vi "Common_DoesClassExist.vi"(1 "ClassPath":path, 2 "ClassName":string) -> (15 "ClassExists":bool, 16 "llb-class":bool, 17 "llb/LvCLass-Path":path, 18 "LvClassExists":bool)   [LabVIEW 2020]
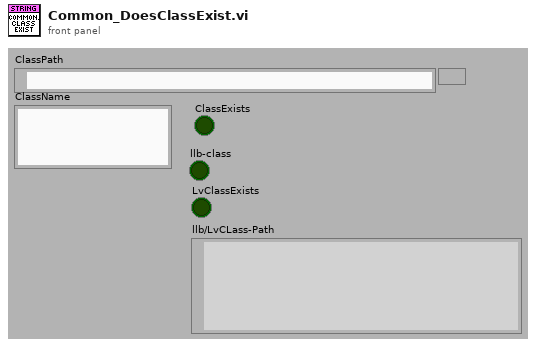
[diagram p1: front panel]
types:
  T1 = typedef "Librarian File Info Out.ctl" = cluster{"creation date":u32, "last mod date":u32, "type":string, "creator":string, "LV version":i32, "size":i32, "top level":bool}
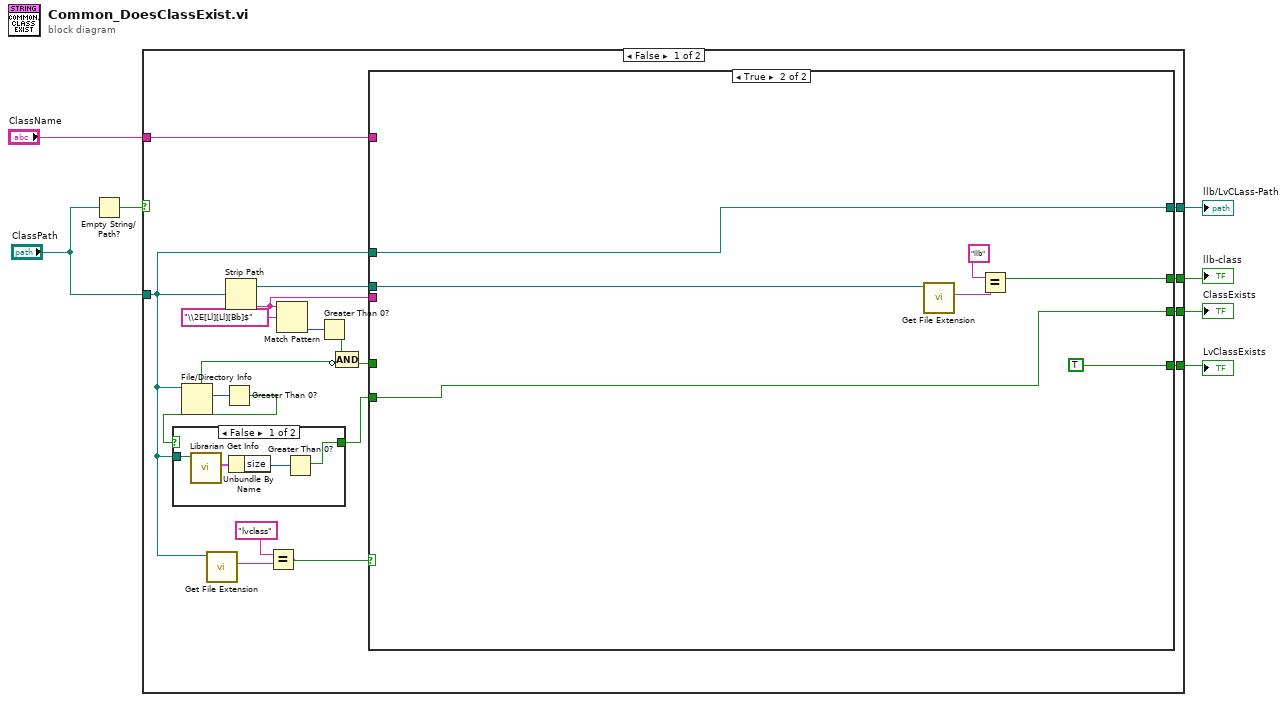
[diagram p0: block diagram]
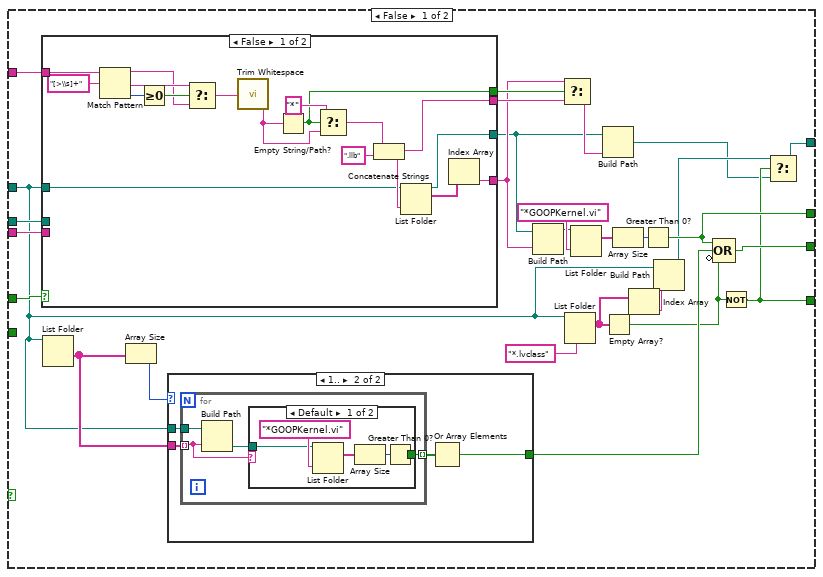
[diagram p3: hidden frame]
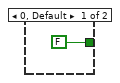
[diagram p4: hidden frame]
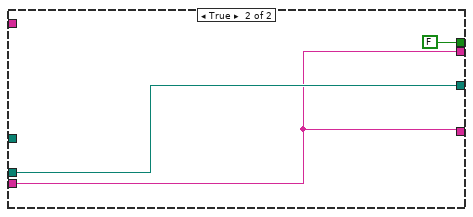
[diagram p6: hidden frame]
diagram:
  n1 = Empty String/Path?(string/path="ClassPath") -> (empty?=w1:bool)
  n2 = case shown="False" w1 {
    tunnel: [w26 _] -> w7
    tunnel: [w25 _] -> w6
    tunnel: "ClassName" -> [w24 _]
    tunnel: [w23 _] -> w4
    tunnel: [w13 _] -> w3
    tunnel: "ClassPath" -> [w11 _]
    frame False {
      n3 = File/Directory Info(path=w11) -> (directory=w10:bool, size=w12:i64)  [unwired: 1 in, 5 out]
      n4 = call <vilib>:"Get File Extension.vi"("file"=w11) -> ("lowercase file extension"=w16:string)  [unwired: 1 in, 9 out]
      n5 = Greater Than 0?(x=w12) -> (x > 0?=w9:bool)
      n6 = case shown="False" w9 {
        selector: w9 -> [_ w31]
        tunnel: w11 -> [w28 _]
        tunnel: [w27 w31] -> w8
        frame False {
          n7 = call <vilib>:"Librarian Get Info.vi"("path"=w28) -> ("file information"=w30:T1)  [unwired: 1 in, 9 out]
          n8 = Unbundle By Name(w30) -> ("size"=w29:i32)
          n9 = Greater Than 0?(x=w29) -> (x > 0?=w27:bool)
        }
        frame True {
        }
      }
      n10 = Strip Path(path=w11) -> (stripped path=w18:path, name=w17:string)
      n11 = Equal?(x="lvclass", y=w16) -> (x = y?=w14:bool)
      n12 = Match Pattern(string=w17, regular expression="\\2E[Ll][Ll][Bb]$") -> (offset past match=w21:i32)  [unwired: 4 out]
      n13 = Greater Than 0?(x=w21) -> (x > 0?=w20:bool)
      n14 = Compound Arithmetic op=AND(w20, invert w10) -> (w19:bool)
      n15 = case shown="True" w14 {
        tunnel: [w40 w95] -> w26
        tunnel: [w32 w93] -> w25
        tunnel: w24 -> [w58 _]
        tunnel: [w48 w96] -> w23
        tunnel: w19 -> [w47 _]
        tunnel: w18 -> [w46 w94]
        tunnel: w17 -> [w45 _]
        tunnel: w11 -> [w36 w93]
        tunnel: [w35 TRUE] -> w13
        tunnel: w8 -> [_ w95]
        frame False {
          n16 = case shown="False" w47 {
            tunnel: w58 -> [w80 _]
            tunnel: [w78 FALSE] -> w57
            tunnel: [w77 w90] -> w56
            tunnel: [w75 w91] -> w42
            tunnel: [w74 w90] -> w50
            tunnel: w36 -> [w73 _]
            tunnel: w46 -> [_ w91]
            tunnel: w45 -> [_ w90]
            frame False {
              n17 = Match Pattern(string=w80, regular expression="[>\\s]+") -> (before substring=w82:string, after substring=w84:string, offset past match=w85:i32)  [unwired: 2 out]
              n18 = Greater Or Equal To 0?(x=w85) -> (x >= 0?=w83:bool)
              n19 = Select(t=w84, s=w83, f=w82) -> (s? t:f=w81:string)
              n20 = call <vilib>:"Trim Whitespace.vi"("string"=w81) -> ("trimmed string"=w79:string)  [unwired: 1 in]
              n21 = Empty String/Path?(string/path=w79) -> (empty?=w78:bool)
              n22 = Select(t="*", s=w78, f=w79) -> (s? t:f=w88:string)
              n23 = Concatenate Strings(w88, ".llb" ("string")) -> (w77:string)
              n24 = List Folder(path=w73, pattern=w77) -> (path out=w75:path, filenames=w76:string[])  [unwired: 1 in, 3 out]
              n25 = Index Array(array=w76) -> (element=w74:string)  [unwired: 1 in]
            }
            frame True {
            }
          }
          n26 = List Folder(path=w36) -> (folder names=w54:string[])  [unwired: 1 in, 5 out]
          n27 = Array Size(array=w54) -> (size(s)=w44:i32)
          n28 = case shown="1.." w44 {
            tunnel: w54 -> [_ w63]
            tunnel: [FALSE w61] -> w43
            tunnel: w36 -> [_ w60]
            frame 0, Default {
            }
            frame 1.. {
              n29 = for {
                tunnel: w63 -> [w66] mode=indexing
                tunnel: w60 -> [w67]
                tunnel: [w64] -> w62 mode=indexing
                n30 = Build Path(base path=w67, name or relative path=w66) -> (appended path=w65:path)
                n31 = case shown="Default" w66 {
                  tunnel: w65 -> [w69 _]
                  tunnel: [w68 _] -> w64
                  frame Default {
                    n32 = List Folder(path=w69, pattern="*GOOPKernel.vi") -> (filenames=w71:string[])  [unwired: 1 in, 4 out]
                    n33 = Array Size(array=w71) -> (size(s)=w72:i32)
                    n34 = Greater Than 0?(x=w72) -> (x > 0?=w68:bool)
                  }
                  frame "Demo", "Example", "Examples", "Test" {
                  }
                }
              }
              n35 = Or Array Elements(Boolean array=w62) -> (logical OR=w61:bool)
            }
          }
          n36 = Build Path(base path=w42, name or relative path=w50) -> (appended path=w49:path)
          n37 = Select(t=w50, s=w57, f=w56) -> (s? t:f=w55:string)
          n38 = List Folder(path=w36, pattern="*.lvclass") -> (filenames=w38:string[])  [unwired: 1 in, 4 out]
          n39 = List Folder(path=w49, pattern="*GOOPKernel.vi") -> (filenames=w52:string[])  [unwired: 1 in, 4 out]
          n40 = Build Path(base path=w42, name or relative path=w55) -> (appended path=w33:path)
          n41 = Empty Array?(array=w38) -> (empty?=w39:bool)
          n42 = Array Size(array=w52) -> (size(s)=w51:i32)
          n43 = Index Array(array=w38) -> (element=w37:string)  [unwired: 1 in]
          n44 = Greater Than 0?(x=w51) -> (x > 0?=w48:bool)
          n45 = Build Path(base path=w36, name or relative path=w37) -> (appended path=w34:path)
          n46 = Compound Arithmetic op=OR(w48, w43, invert w39) -> (w40:bool)
          n47 = Not(x=w39) -> (.not. x?=w35:bool)
          n48 = Select(t=w34, s=w35, f=w33) -> (s? t:f=w32:path)
        }
        frame True {
          n49 = call <vilib>:"Get File Extension.vi"("file"=w94) -> ("lowercase file extension"=w97:string)  [unwired: 1 in, 9 out]
          n50 = Equal?(x="llb", y=w97) -> (x = y?=w96:bool)
        }
      }
    }
    frame True {
    }
  }
  "ClassExists" <- w7
  "llb-class" <- w4
  "llb/LvCLass-Path" <- w6
  "LvClassExists" <- w3
